vi "View Detailed Histogram.vi"(1 "LSB/FS":bool, 2 "X":waveform(dbl)[](array[waveform])) -> ()   [LabVIEW 2014]
uses:
  <vilib>/Analysis/NI_AALPro.lvlib
panel:
  out "Hist Type":string
  out "FS Histogram":T1(graph)
  out "LSB Histogram":T1(graph)
  in  "Close VI":bool
  out "Signal Preview":waveform(dbl)[](graph)
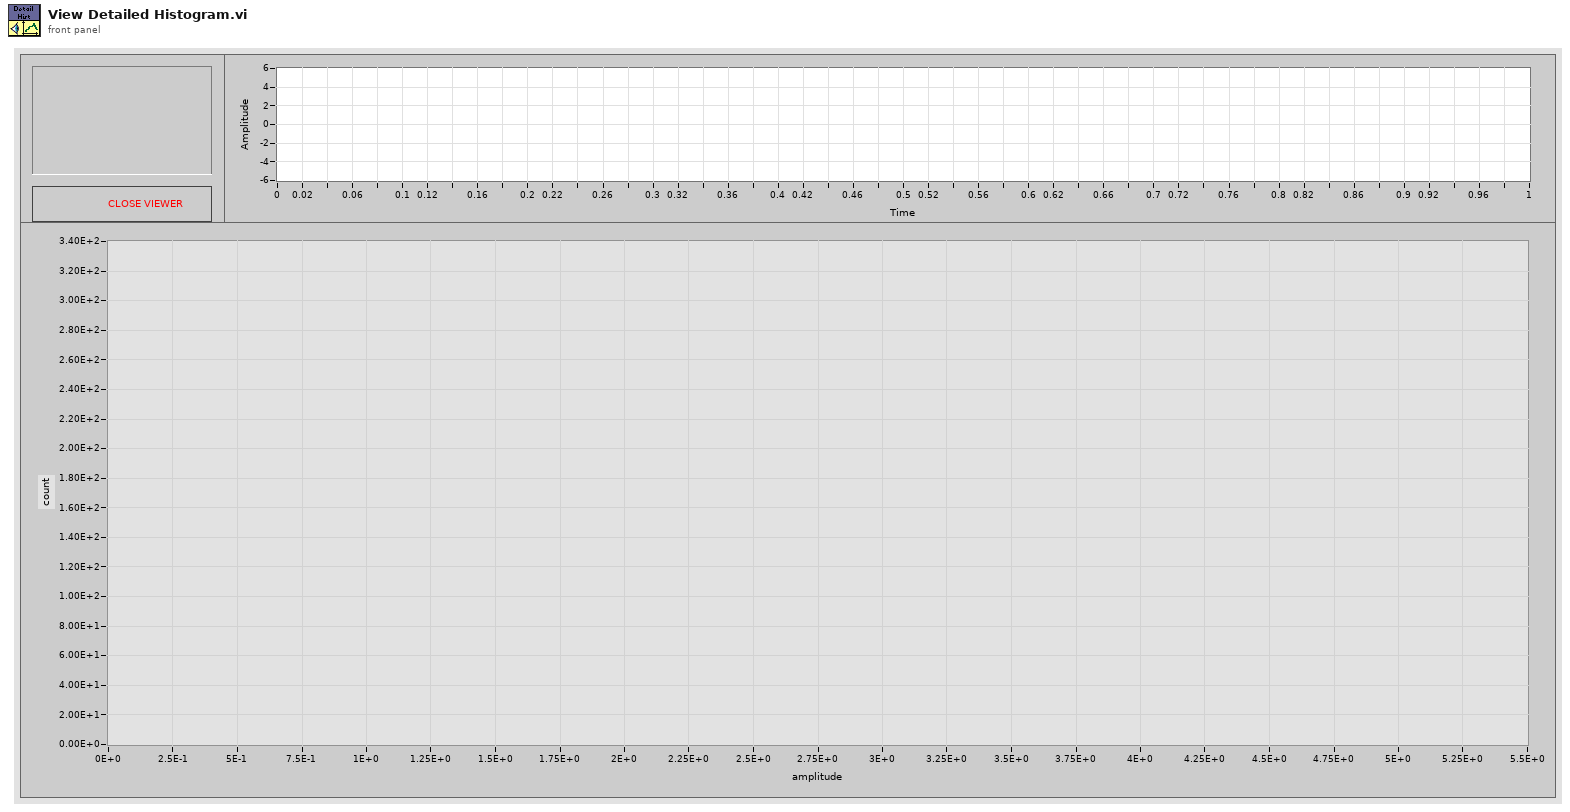
[diagram p1: front panel]
types:
  T1 = cluster{"X Values":dbl[], "Histogram: h(x)":i32[]}
  T2 = enum16{"Always On", "Always Off", "Off While Running"}
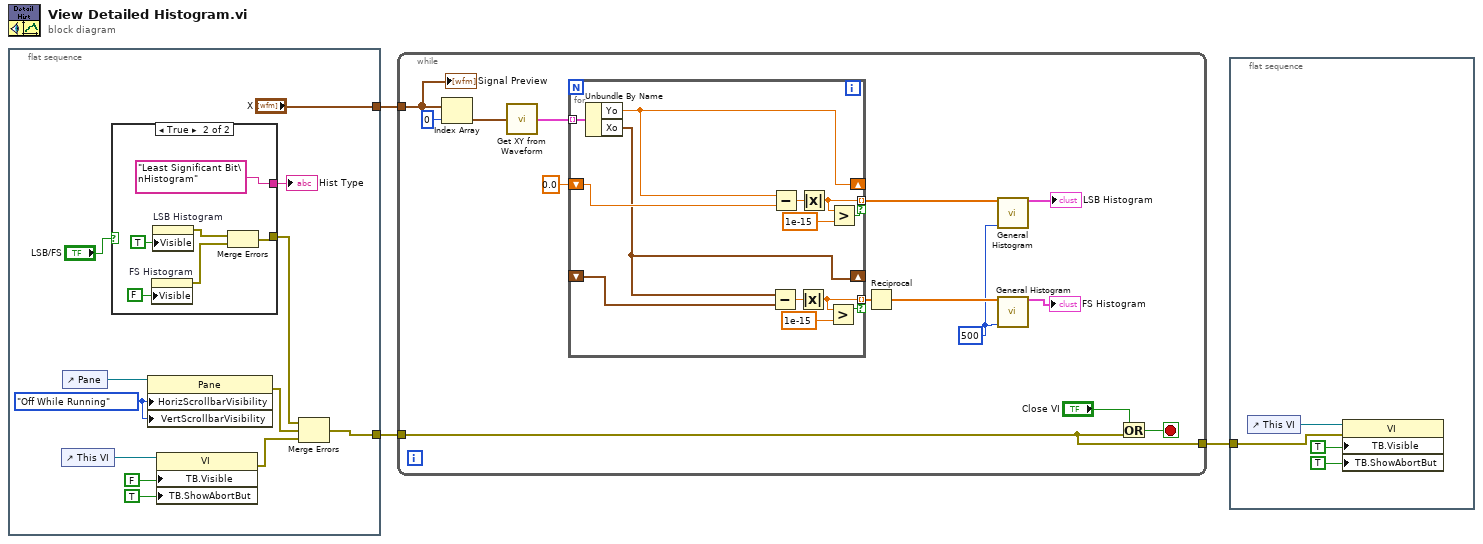
[diagram p0: block diagram]
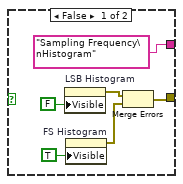
[diagram p2: hidden frame]
diagram:
  n1 = flat-sequence {
    tunnel: ["X"] -> w3
    tunnel: [w7] -> w2
    frame #0 {
      w13 = T2."Off While Running" ("Horizontal Scrollbar Visibility")
      n2 = control-ref of="This VI"() -> (w12:refnum<vi>)
      n3 = control-ref of="Pane"() -> (w14:refnum<vi>)
      n4 = case shown="True" "LSB/FS" {
        tunnel: [w17 w23] -> w5
        tunnel: ["Sampling Frequency\nHistogram" "Least Significant Bit\nHistogram"] -> w4
        frame False {
          n5 = property on="LSB Histogram" class="XYGraph (strict)"("Visible"=FALSE) -> (error out=w20:errorcluster)  [unwired: 2 in, 1 out]
          n6 = property on="FS Histogram" class="XYGraph (strict)"("Visible"=TRUE) -> (error out=w18:errorcluster)  [unwired: 2 in, 1 out]
          n7 = Merge Errors(w20, w18) -> (w17:errorcluster)
        }
        frame True {
          n8 = property on="FS Histogram" class="XYGraph (strict)"("Visible"=FALSE) -> (error out=w25:errorcluster)  [unwired: 2 in, 1 out]
          n9 = property on="LSB Histogram" class="XYGraph (strict)"("Visible"=TRUE) -> (error out=w24:errorcluster)  [unwired: 2 in, 1 out]
          n10 = Merge Errors(w24, w25) -> (w23:errorcluster)
        }
      }
      "Hist Type" <- w4
      n11 = property class="Pane"(reference=w14, "HorizScrollbarVisibility"=w13, "VertScrollbarVisibility"=w13) -> (error out=w8:errorcluster)  [unwired: 1 in, 1 out]
      n12 = property class="VI"(reference=w12, "TB.Visible"=FALSE ("Tool Bar:Visible"), "TB.ShowAbortBut"=TRUE ("Tool Bar:Visible")) -> (error out=w9:errorcluster)  [unwired: 1 in, 1 out]
      n13 = Merge Errors(w5, w8, w9) -> (w7:errorcluster)
    }
  }
  n14 = while {
    tunnel: w3 -> [w33]
    tunnel: w2 -> [w30]
    tunnel: [w30] -> w1
    stop <- w31 stop-if-true
    w28 = 500 ("# bins")
    n15 = Index Array(array=w33, index=0) -> (element=w36:waveform(dbl))
    n16 = call "Get XY from Waveform.vi"("Waveform In"=w36) -> ("XY Array Out"=w39:cluster{"Yo":dbl, "Xo":timestamp}[])
    n17 = for {
      tunnel: [w45] -> w41 mode=indexing if=w53
      tunnel: w39 -> [w52] mode=indexing
      shift-right: [w50] -> _
      shift-left: 0.0 ("Yo") -> [w51]
      shift-right: [w48] -> _
      shift-left: _ -> [w47]
      tunnel: [w43] -> w37 mode=indexing if=w46
      n18 = Unbundle By Name(w52) -> ("Yo"=w50:dbl, "Xo"=w48:timestamp)
      n19 = Subtract(x=w48, y=w47) -> (x-y=w49:dbl)
      n20 = Subtract(x=w50, y=w51) -> (x-y=w54:dbl)
      n21 = Absolute Value(x=w49) -> (abs(x)=w43:dbl)
      n22 = Absolute Value(x=w54) -> (abs(x)=w45:dbl)
      n23 = Greater?(x=w43, y=1e-15) -> (0:w46:bool)
      n24 = Greater?(x=w45, y=1e-15) -> (0:w53:bool)
    }
    n25 = Reciprocal(x=w37) -> (1/x=w40:dbl[])
    n26 = call <vilib>:"General Histogram.vi"("X"=w41, "# bins"=w28) -> ("Histogram Graph"=→"LSB Histogram":T1)  [unwired: 9 in, 4 out]
    n27 = call <vilib>:"General Histogram.vi"("X"=w40, "# bins"=w28) -> ("Histogram Graph"=→"FS Histogram":T1)  [unwired: 9 in, 4 out]
    n28 = Or(x="Close VI", y=w30) -> (x .or. y?=w31:bool)
    "Signal Preview" <- w33
  }
  n29 = flat-sequence {
    tunnel: w1 -> [w55]
    frame #0 {
      n30 = control-ref of="This VI"() -> (w56:refnum<vi>)
      n31 = property class="VI"(reference=w56, error in=w55, "TB.Visible"=TRUE ("Tool Bar:Visible"), "TB.ShowAbortBut"=TRUE ("Tool Bar:Visible")) -> ()  [unwired: 2 out]
    }
  }
